vi "Ramp_v2.vi"() -> ()   [LabVIEW 2016]
uses:
  BERTTA.dll
panel:
  in  "time_wait":dbl[](array[numeric])
  in  "Tr":dbl
  in  "Tr_Tj":i32=1
  in  "T_manual":dbl=20.0
  out "T0_":dbl
  out "elapsed":dbl
  out "step":dbl
  out "Waveform Chart":dynamicdata(graph)
  in  "port":i32=1
  in  "T_sp":dbl[](array[numeric])
  in  "time_set":dbl[](array[numeric])
  in  "manual":i32
  in  "enable":i32
  in  "reset":i32
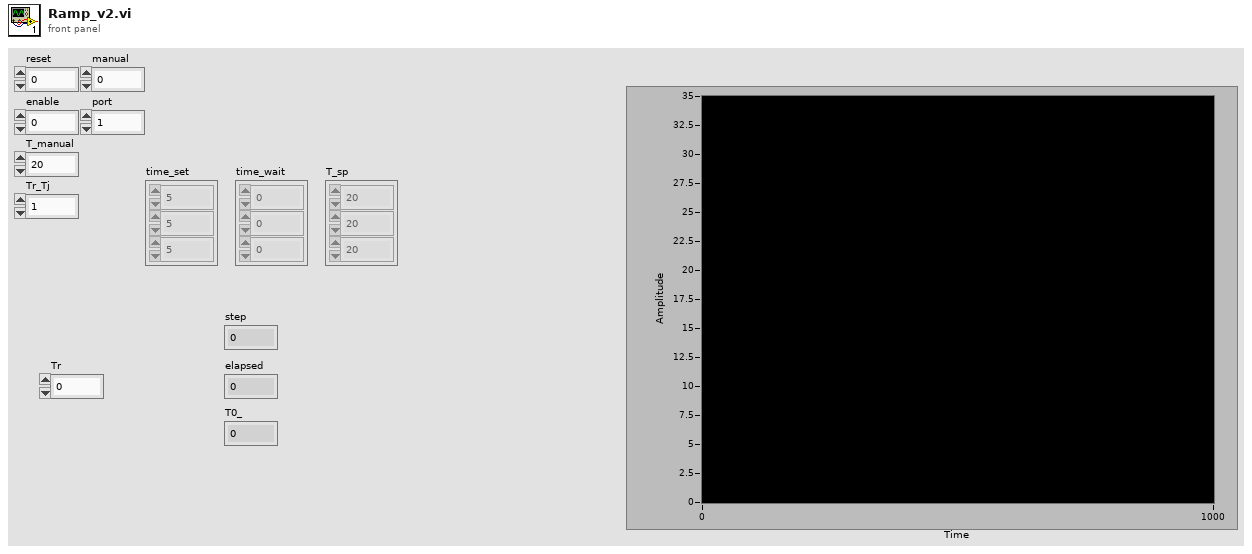
[diagram p1: front panel]
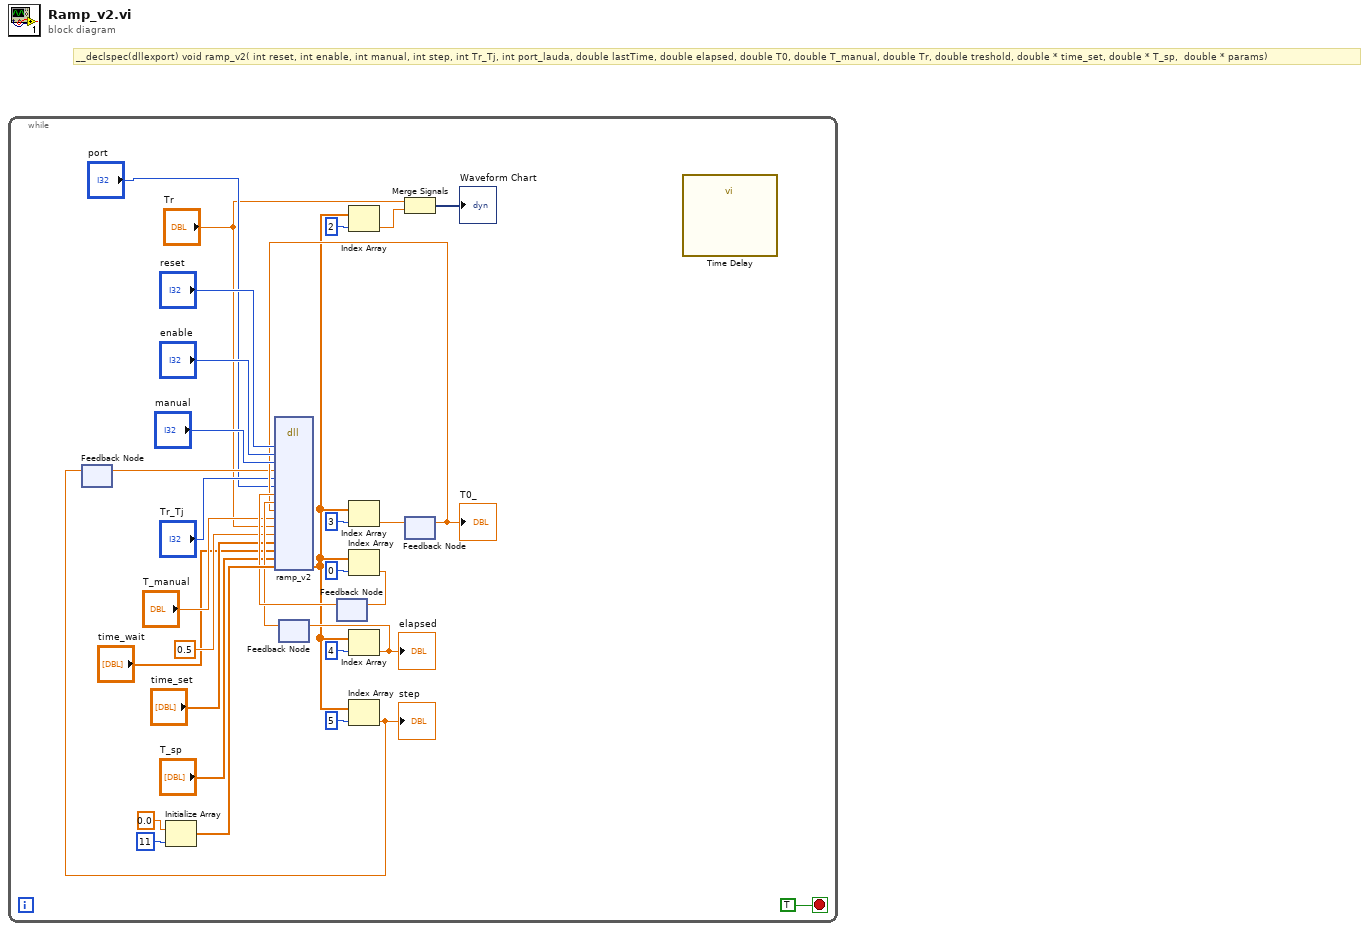
[diagram p0: block diagram]
diagram:
  # "__declspec(dllexport) void ramp_v2( int reset, int enable, int manual, int step, int Tr_Tj, int port_lauda, double lastTime, double elapsed, double T0, double T_manual, double Tr, double treshold, double * time_set, double * T_sp,  double * params)"
  n1 = while {
    stop <- TRUE stop-if-true
    n2 = feedback #1() -> (w11:dbl)  [unwired: 1 in]
    n3 = Initialize Array(0.0 ("element"), 11 ("dimension size")) -> (w26:dbl[])
    n4 = feedback #2() -> (w20:dbl)  [unwired: 1 in]
    n5 = feedback #3() -> (w23:dbl)  [unwired: 1 in]
    n6 = feedback #4() -> (w17:dbl)  [unwired: 1 in]
    "T0_" <- w17
    n7 = dll-call lib="C:/Users/shresplab/OneDrive - Kemira Oyj/Documents/GitHub/Bertta/BERTTA/x64/Debug/BERTTA.dll" fn="ramp_v2"("reset"="reset", "enable"="enable", "manual"="manual", "step"=w11, "Tr_Tj"="Tr_Tj", "port_lauda"="port", "lastTime"=w23, "elapsed"=w20, "T0"=w17, "T_manual"="T_manual", "Tr"="Tr", "treshold"=0.5, "time_set"="time_set", "time_wait"="time_wait", "T_sp"="T_sp", "params"=w26) -> ("params"=w9:dbl[])  [unwired: 19 in, 2 out]
    n8 = Index Array(array=w9, index=2) -> (element=w7:dbl)
    n9 = Index Array(array=w9, index=3) -> (element=w18:dbl)
    n10 = Index Array(array=w9, index=0) -> (element=w24:dbl)
    n11 = feedback-in #3(w24) -> ()
    n12 = Index Array(array=w9, index=4) -> (element=w21:dbl)
    "elapsed" <- w21
    n13 = feedback-in #2(w21) -> ()
    n14 = Index Array(array=w9, index=5) -> (element=w12:dbl)
    "step" <- w12
    n15 = feedback-in #1(w12) -> ()
    n16 = Merge Signals("Tr", w7) -> (→"Waveform Chart":dynamicdata)
    n17 = feedback-in #4(w18) -> ()
    n18 = call "Time Delay"() -> ()  [unwired: 11 in, 1 out]
  }
